vi "libssh2_sftp_closedir.vi"(8 "error in (no error)":errorcluster, 11 "sftp handle":T1) -> (0 "error out":errorcluster)   [LabVIEW 2013, in "libssh2.lvlib"]
doc: "Close a directory handle."
uses:
  libssh2.lvlib
  SFTP Handle Refnum.ctl
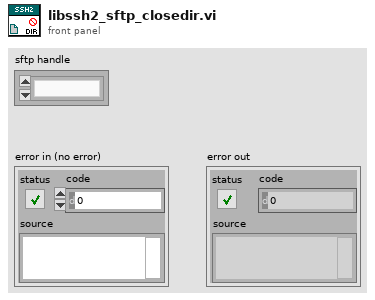
[diagram p1: front panel]
types:
  T1 = typedef "libssh2.lvlib/SFTP Handle Refnum.ctl" = refnum<k1>
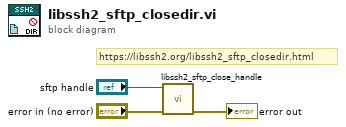
[diagram p0: block diagram]
diagram:
  # "https://libssh2.org/libssh2_sftp_closedir.html"
  n1 = call "libssh2_sftp_close_handle.vi"("error in (no error)"="error in (no error)", "sftp handle"="sftp handle") -> ("error out"=→"error out":errorcluster)  [unwired: 9 in]
